vi "En-queue RT torque data element.vi"(9 "Torque data":dbl[](array[numeric]), 11 "RT Queues":T1) -> (1 "timed out?":bool)   [LabVIEW 2018]
uses:
  Type Defs/Queues cluster.ctl
  ICL-LabVIEW_General/Message Scheduler/message scheduler.lvclass
panel:
  out "RT Queues out":T1
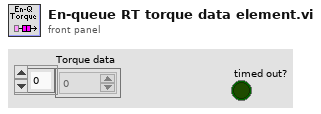
[diagram p1: front panel]
types:
  T1 = typedef "Queues cluster.ctl" = cluster{"RT Message":refnum<queue>, "RT Comms":refnum<queue>, "RT Data":refnum<queue>, "RT FIFO":refnum<queue>, "message scheduler":refnum<class "message scheduler.lvclass">}
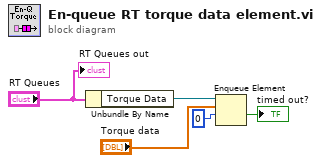
[diagram p0: block diagram]
diagram:
  n1 = Unbundle By Name("RT Queues") -> ("Torque Data"=w4:refnum<queue>)
  n2 = Enqueue Element(queue=w4, element="Torque data", timeout in ms (-1)=0) -> (timed out?=→"timed out?":bool)  [unwired: 1 in, 2 out]
  "RT Queues out" <- "RT Queues"
